vi "Begin.vi"(8 "error in":errorcluster) -> (0 "error out":errorcluster)   [LabVIEW 2019]
doc: "Called before other user functions, this VI is expected to open initial I/O refnums, load in file data, and do all program initialization. Notice that the <B>error out</B> terminal is simply used for data flow. Wiring it to other structures or subVIs ensures that this VI runs first."
uses:
  <vilib>/Rock Robotics/WPI/DriverStation/WPI_DriverStationRobotMode2.ctl
  <vilib>/Rock Robotics/WPI/Joystick/WPI_JoystickDeviceEnum.ctl
  <vilib>/Rock Robotics/WPI/SafetyOutput/WPI_SafetyOutputConfigMenu.ctl
  <vilib>/Rock Robotics/WPI/ThirdParty/REV Robotics/SPARK MAX/Typedef/Spark MAX Motor Type.ctl
  <vilib>/Rock Robotics/WPI/ThirdParty/REV Robotics/SPARK MAX/Typedef/Spark MAX Sensor Type.ctl
  <vilib>/Rock Robotics/WPI/ThirdParty/Phoenix-LabVIEW/Motor Controller/Controls/CTRE_Phoenix_MotorControl_FeedbackDevice.ctl
  <vilib>/Rock Robotics/SystemInterfaces/DIO/FPGA_DIOPWMChannel.ctl
  Robot Global Data.vi
  <vilib>/Rock Robotics/Network Tables/NT Write String Array.vi
  <vilib>/Rock Robotics/Network Tables/NT Write Number.vi
  Refnums.vi
  CAN_ID.vi
  <vilib>/Rock Robotics/WPI/RobotDrive/WPI_RobotDriveOpen2MotorWithExistingMotors.vi
  PID.vi
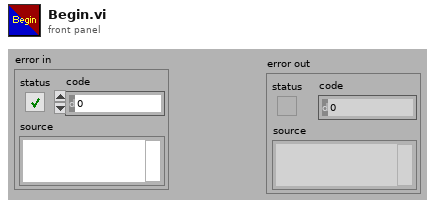
[diagram p1: front panel]
types:
  T1 = typedef "WPI_DriverStationRobotMode2.ctl" = enum16{"Autonomous Disabled", "Autonomous Enabled", "Teleop Disabled", "Teleop Enabled", "Disconnected", "Finish", "Test Disabled", "Test Enabled", "Emergency Stopped"}
  T2 = typedef "WPI_JoystickDeviceEnum.ctl" = enum16{"USB 0", "USB 1", "USB 2", "USB 3", "USB 4", "USB 5"}
  T3 = typedef "WPI_SafetyOutputConfigMenu.ctl" = enum16{"Enable", "Disable"}
  T4 = typedef "FPGA_DIOPWMChannel.ctl" = enum8{"PWM 0", "PWM 1", "PWM 2", "PWM 3", "PWM 4", "PWM 5", "PWM 6", "PWM 7", "PWM 8", "PWM 9", "PWM MXP 0", "PWM MXP 1", "PWM MXP 2", "PWM MXP 3", "PWM MXP 4", "PWM MXP 5", "PWM MXP 6", "PWM MXP 7", "PWM MXP 8", "PWM MXP 9", "Invalid"}
  T5 = typedef "WPI_JoystickDevRef.ctl" = cluster{"Device":T2}
  T6 = typedef "Spark MAX Sensor Type.ctl" = enum16{"No Sensor", "Hall Sensor", "Encoder", "-Not Available-", "Analog", "Alternate Encoder"}
  T7 = typedef "Spark MAX Motor Type.ctl" = enum16{"Brushed", "Brushless"}
  T8 = typedef "WPI_MotorControlDeviceRef.ctl" = cluster{"DeviceStatus":errorcluster, "Type":T9, "PWM":cluster{"PWM Channel":T4, "DeadBand":T10}, "CAN":cluster{"Device Number":u8, "SetOutput VI Ref":variant, "GetOutput VI Ref":variant, "Enable VI Ref":variant, "Disable VI Ref":variant, "Data":variant}, "Invert":bool, "DIO PWM":cluster{"PWM \"Enable\" Channel":T4, "DIOChannel":T11, "PWM Rate":dbl}}
  T9 = typedef "WPI_MotorControlType.ctl" = enum16{"PWM", "CAN", "DIO PWM"}
  T10 = typedef "WPI_PWMDeadband.ctl" = cluster{"Name":string, "maxPositivePwm":i32, "minPositivePwm":i32, "centerPwm":i32, "maxNegativePwm":i32, "minNegativePwm":i32, "angularRange":u16}
  T11 = typedef "FPGA_DIOChannel.ctl" = enum8{"DIO 0", "DIO 1", "DIO 2", "DIO 3", "DIO 4", "DIO 5", "DIO 6", "DIO 7", "DIO 8", "DIO 9", "DIO MXP 0", "DIO MXP 1", "DIO MXP 2", "DIO MXP 3", "DIO MXP 4", "DIO MXP 5", "DIO MXP 6", "DIO MXP 7", "DIO MXP 8", "DIO MXP 9", "DIO MXP 10", "DIO MXP 11", "DIO MXP 12", "DIO MXP 13", "DIO MXP 14", "DIO MXP 15", "SPI Port CS1", "SPI Port CS2", "SPI Port CS3", "SPI Port MISO", "SPI Port MOSI", "Invalid"}
  T12 = typedef "WPI_RobotDriveDevRef.ctl" = cluster{"DevStatus":errorcluster, "Motors[]":T8[], "Square Inputs":bool, "Max Output":dbl}
  T13 = typedef "CTRE_Phoenix_MotorControl_FeedbackDevice.ctl" = i8
  T14 = cluster{"P":dbl, "I":dbl, "D":dbl, "F":dbl, "I Zone":dbl}
  T15 = typedef "WPI_ServoDeviceRef.ctl" = cluster{"DeviceStatus":errorcluster, "PWM Channel":T4, "DeadBand":T10}
  T16 = cluster{"LEFT_FRONT_DRIVE":u8, "LEFT_REAR_DRIVE":u8, "RIGHT_FRONT_DRIVE":u8, "RIGHT_REAR_DRIVE":u8, "TALON":u8}
  T17 = cluster{"NEO_RobotDrive":T12, "TALON_SRX":T8, "RIGHT_DRIVE":T8, "LEFT_DRIVE":T8}
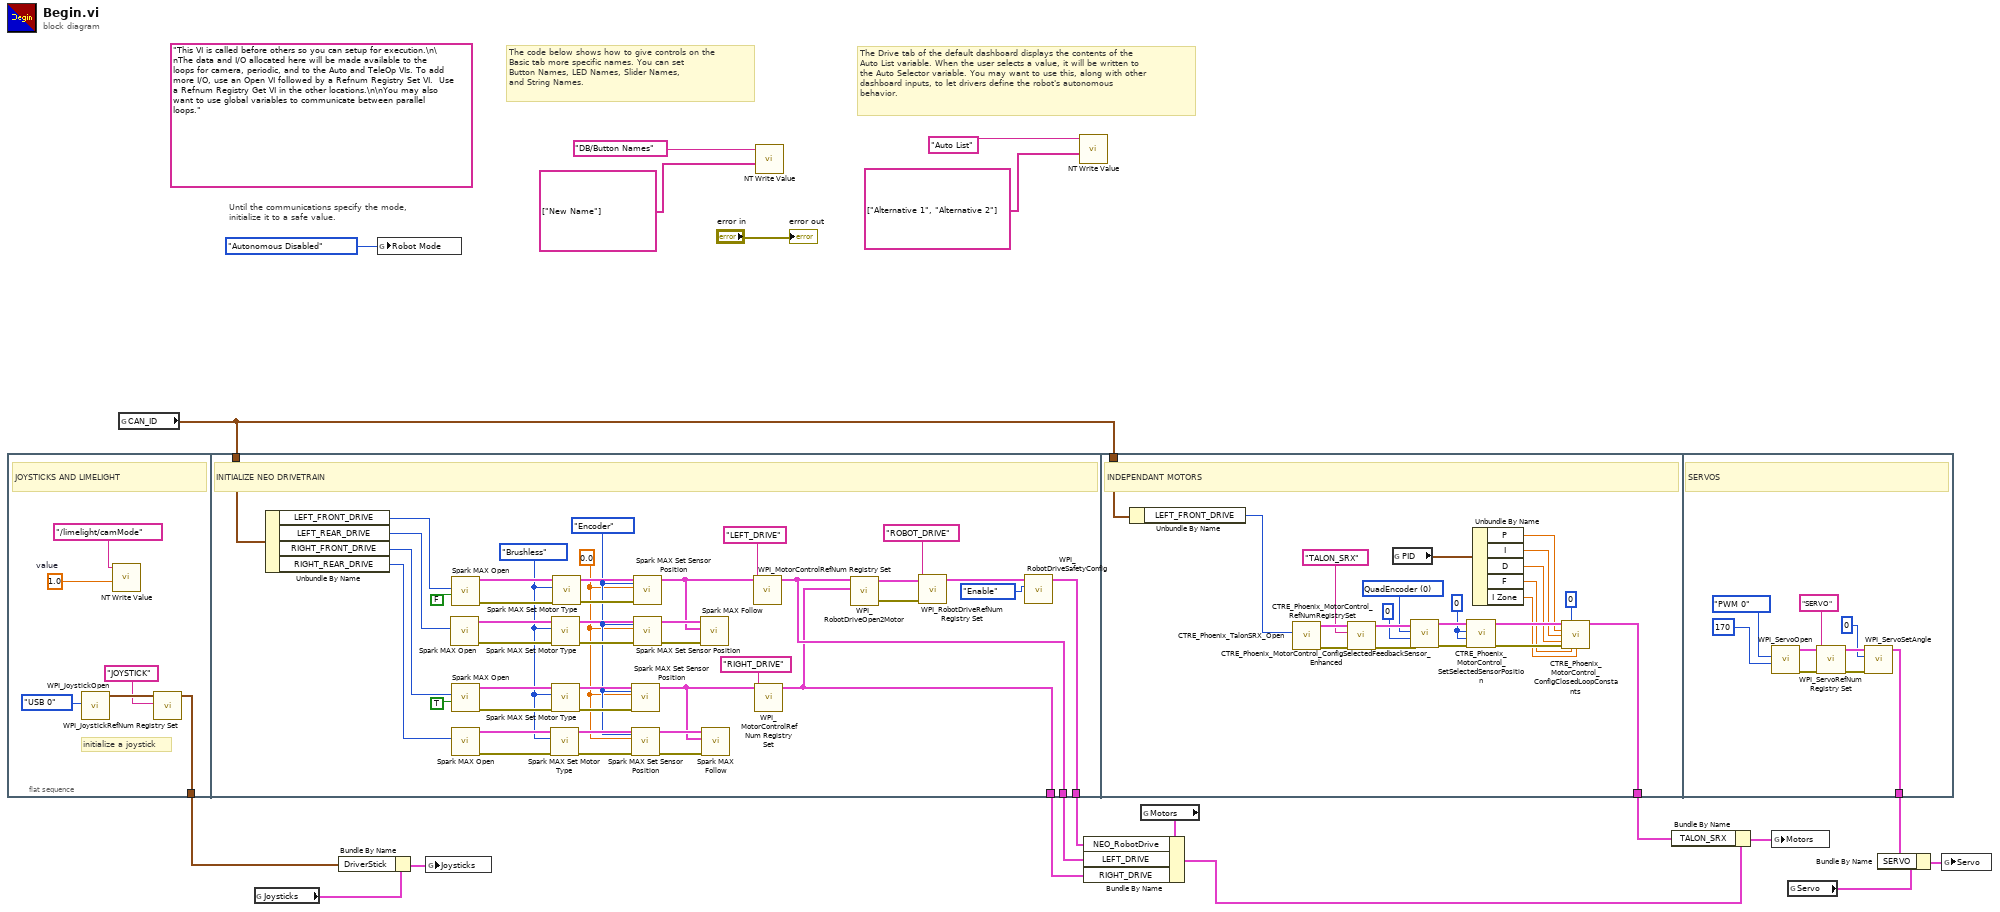
[diagram p0: block diagram]
diagram:
  (unwired) "This VI is called before others so you can setup for execution.\n\nThe data and I/O allocated here will be made available to the loops for camera, periodic, and to the Auto and TeleOp VIs. To add more I/O, use an Open VI followed by a Refnum Registry Set VI.  Use a Refnum Registry Get VI in the other locations.\n\nYou may also want to use global variables to communicate between parallel loops."
  # "The Drive tab of the default dashboard displays the contents of the\nAuto List variable. When the user selects a value, it will be written to\nthe Auto Selector variable. You may want to use this, along with other\ndashboard inputs, to let drivers define the robot's autonomous\nbehavior."
  # "The code below shows how to give controls on the\nBasic tab more specific names. You can set\nButton Names, LED Names, Slider Names,\nand String Names."
  # "Until the communications specify the mode,\ninitialize it to a safe value."
  n1 = flat-sequence {
    tunnel: [w23] -> w13
    tunnel: [w40] -> w6
    tunnel: w8 -> [w37]
    tunnel: [w28] -> w5
    tunnel: [w27] -> w4
    tunnel: [w71] -> w3
    tunnel: w8 -> [w69]
    tunnel: [w91] -> w10
    frame #0 {
      w21 = 1.0  # value
      # "initialize a joystick"
      # "JOYSTICKS AND LIMELIGHT"
      n2 = call <vilib>:"WPI_JoystickOpen.vi"("JoystickDevice"=WPI_JoystickDeviceEnum."USB 0") -> ("JoystickDevRef"=w26:T5)  [unwired: 10 in]
      n3 = call-poly <vilib>:"NT Write Value.vi"("Numeric"=w21, "Name"="/limelight/camMode") -> ()  [unwired: 9 in, 1 out]
      n4 = call <vilib>:"WPI_JoystickRefNum Registry Set.vi"("refnum name"="JOYSTICK", "JoystickDevRef"=w26) -> ("JoystickDevRef"=w23:T5)  [unwired: 8 in, 1 out]
    }
    frame #1 {
      w44 = 0.0 ("Position")
      w45 = Spark_MAX_Sensor_Type."Encoder" ("Sensor Type (Hall Sensor)")
      w43 = Spark_MAX_Motor_Type."Brushless" ("Motor Type")
      # "INITIALIZE NEO DRIVETRAIN"
      n5 = Unbundle By Name(w37) -> ("LEFT_FRONT_DRIVE"=w36:u8, "LEFT_REAR_DRIVE"=w35:u8, "RIGHT_FRONT_DRIVE"=w34:u8, "RIGHT_REAR_DRIVE"=w33:u8)
      n6 = call <vilib>:"Spark MAX Open.vi"("Device Number"=w35) -> ("error out"=w50:errorcluster, "MotorControlDeviceRef"=w49:T8)  [unwired: 9 in]
      n7 = call <vilib>:"Spark MAX Open.vi"("Invert"=FALSE, "Device Number"=w36) -> ("error out"=w48:errorcluster, "MotorControlDeviceRef"=w47:T8)  [unwired: 8 in]
      n8 = call <vilib>:"Spark MAX Open.vi"("Invert"=TRUE, "Device Number"=w34) -> ("error out"=w53:errorcluster, "MotorControlDeviceRef"=w54:T8)  [unwired: 8 in]
      n9 = call <vilib>:"Spark MAX Open.vi"("Device Number"=w33) -> ("error out"=w52:errorcluster, "MotorControlDeviceRef"=w51:T8)  [unwired: 9 in]
      n10 = call <vilib>:"Spark MAX Set Motor Type.vi"("error in (no error)"=w52, "Motor Type"=w43, "MotorControlDevRef"=w51) -> ("error out"=w62:errorcluster, "MotorControlDeviceRef"=w61:T8)  [unwired: 7 in]
      n11 = call <vilib>:"Spark MAX Set Motor Type.vi"("error in (no error)"=w50, "Motor Type"=w43, "MotorControlDevRef"=w49) -> ("error out"=w58:errorcluster, "MotorControlDeviceRef"=w57:T8)  [unwired: 7 in]
      n12 = call <vilib>:"Spark MAX Set Motor Type.vi"("error in (no error)"=w53, "Motor Type"=w43, "MotorControlDevRef"=w54) -> ("error out"=w60:errorcluster, "MotorControlDeviceRef"=w59:T8)  [unwired: 7 in]
      n13 = call <vilib>:"Spark MAX Set Motor Type.vi"("error in (no error)"=w48, "Motor Type"=w43, "MotorControlDevRef"=w47) -> ("error out"=w56:errorcluster, "MotorControlDeviceRef"=w55:T8)  [unwired: 7 in]
      n14 = call <vilib>:"Spark MAX Set Sensor Position.vi"("Sensor Type (Hall Sensor)"=w45, "error in"=w60, "Position"=w44, "MotorControlDeviceRef"=w59) -> ("MotorControlDeviceRef"=w32:T8)  [unwired: 6 in, 1 out]
      n15 = call <vilib>:"Spark MAX Set Sensor Position.vi"("Sensor Type (Hall Sensor)"=w45, "error in"=w62, "Position"=w44, "MotorControlDeviceRef"=w61) -> ("error out"=w66:errorcluster, "MotorControlDeviceRef"=w65:T8)  [unwired: 6 in]
      n16 = call <vilib>:"Spark MAX Set Sensor Position.vi"("Sensor Type (Hall Sensor)"=w45, "error in"=w56, "Position"=w44, "MotorControlDeviceRef"=w55) -> ("MotorControlDeviceRef"=w31:T8)  [unwired: 6 in, 1 out]
      n17 = call <vilib>:"Spark MAX Set Sensor Position.vi"("Sensor Type (Hall Sensor)"=w45, "error in"=w58, "Position"=w44, "MotorControlDeviceRef"=w57) -> ("error out"=w63:errorcluster, "MotorControlDeviceRef"=w64:T8)  [unwired: 6 in]
      n18 = call <vilib>:"Spark MAX Follow.vi"("error in (no error)"=w63, "Master Controller"=w31, "MotorControlDeviceRef"=w64) -> ()  [unwired: 7 in, 2 out]
      n19 = call <vilib>:"Spark MAX Follow.vi"("error in (no error)"=w66, "Master Controller"=w32, "MotorControlDeviceRef"=w65) -> ()  [unwired: 7 in, 2 out]
      n20 = call <vilib>:"WPI_MotorControlRefNum Registry Set.vi"("refnum name"="LEFT_DRIVE", "MotorControlDevRef"=w31) -> ("MotorControlDevRef"=w28:T8)  [unwired: 8 in, 1 out]
      n21 = call <vilib>:"WPI_MotorControlRefNum Registry Set.vi"("refnum name"="RIGHT_DRIVE", "MotorControlDevRef"=w32) -> ("MotorControlDevRef"=w27:T8)  [unwired: 8 in, 1 out]
      n22 = call-poly <vilib>:"WPI_RobotDriveOpen2Motor.vi"("Right Motor Dev Ref"=w27, "Left Motor Dev Ref"=w28) -> ("error out"=w68:errorcluster, "RobotDriveDevRef"=w67:T12)  [unwired: 3 in, 5 out]
      n23 = call <vilib>:"WPI_RobotDriveRefNum Registry Set.vi"("error in (no error)"=w68, "refnum name"="ROBOT_DRIVE", "RobotDriveDevRef"=w67) -> ("RobotDriveDevRef"=w46:T12)  [unwired: 1 in, 7 out]
      n24 = call <vilib>:"WPI_RobotDriveSafetyConfig.vi"("mode"=WPI_SafetyOutputConfigMenu."Enable", "RobotDriveDevRef"=w46) -> ("RobotDriveDevRef"=w40:T12)  [unwired: 8 in, 1 out]
    }
    frame #2 {
      w81 = 0 ("New Sensor Position")
      w85 = T13 0 items=["QuadEncoder"=0, "Analog"=2, "Tachometer"=4, "Pulse Width Encoded Position"=8, "Sensor Sum (S0 + S1)"=9, "Sensor Difference (D0 - D1)"=10, "Remote Source 0"=11, "Remote Source 1"=12, "Software Emulated"=15] ("Feedback Device")
      # "INDEPENDANT MOTORS"
      n25 = Unbundle By Name(w69) -> ("LEFT_FRONT_DRIVE"=w70:u8)
      n26 = call <vilib>:"CTRE_Phoenix_TalonSRX_Open.vi"("Device Number"=w70) -> ("error out"=w90:errorcluster, "CAN Talon SRX Ref"=w89:T8)  [unwired: 9 in]
      n27 = call <vilib>:"CTRE_Phoenix_MotorControl_RefNumRegistrySet.vi"("error in (no error)"=w90, "refnum name"="TALON_SRX", "PhoenixMotorControlDevRef"=w89) -> ("error out"=w87:errorcluster, "PhoenixMotorControlDevRef"=w86:T8)  [unwired: 7 in]
      n28 = global read "PID.vi" "PID"() -> (w78:T14)
      n29 = call <vilib>:"CTRE_Phoenix_MotorControl_ConfigSelectedFeedbackSensor_Enhanced.vi"("error in (no error)"=w87, "pidLoopIdx"=0, "Feedback Device"=w85, "PhoenixMotorControlDevRef"=w86) -> ("error out"=w83:errorcluster, "PhoenixMotorControlDevRef"=w82:T8)  [unwired: 6 in]
      n30 = call <vilib>:"CTRE_Phoenix_MotorControl_SetSelectedSensorPosition.vi"("error in (no error)"=w83, "pidLoopIdx"=w81, "New Sensor Position"=w81, "PhoenixMotorControlDevRef"=w82) -> ("error out"=w79:errorcluster, "PhoenixMotorControlDevRef"=w80:T8)  [unwired: 6 in]
      n31 = Unbundle By Name(w78) -> ("P"=w77:dbl, "I"=w76:dbl, "D"=w75:dbl, "F"=w74:dbl, "I Zone"=w73:dbl)
      n32 = call <vilib>:"CTRE_Phoenix_MotorControl_ConfigClosedLoopConstants.vi"("PhoenixMotorControlDevRef"=w80, "slotIdx"=0, "P"=w77, "I"=w76, "D"=w75, "error in (no error)"=w79, "F"=w74, "I Zone"=w73) -> ("PhoenixMotorControlDevRef"=w71:T8)  [unwired: 6 in, 1 out]
    }
    frame #3 {
      # "SERVOS"
      n33 = call <vilib>:"WPI_ServoOpen.vi"("Angular Range"=u16 170, "PWM Channel"=FPGA_DIOPWMChannel."PWM 0") -> ("error out"=w99:errorcluster, "ServoDeviceRef"=w98:T15)  [unwired: 8 in]
      n34 = call <vilib>:"WPI_ServoRefNum Registry Set.vi"("error in (no error)"=w99, "refnum name"="SERVO", "ServoDeviceRef"=w98) -> ("error out"=w95:errorcluster, "ServoDeviceRef"=w94:T15)  [unwired: 7 in]
      n35 = call <vilib>:"WPI_ServoSetAngle.vi"("error in (no error)"=w95, "Angle"=0, "ServoDeviceRef"=w94) -> ("ServoDeviceRef"=w91:T15)  [unwired: 7 in, 1 out]
    }
  }
  n36 = global read "CAN_ID.vi" "CAN_ID"() -> (w8:T16)
  n37 = global read "Refnums.vi" "Joysticks"() -> (w15:cluster{"DriverStick":T5, "OperatorStick":T5})
  n38 = Bundle By Name(cluster=w15, "DriverStick"=w13) -> (w12:cluster{"DriverStick":T5, "OperatorStick":T5})
  n39 = global write "Robot Global Data.vi" "Robot Mode"(WPI_DriverStationRobotMode2."Autonomous Disabled" ("Robot Mode")) -> ()
  n40 = global write "Refnums.vi" "Joysticks"(w12) -> ()
  n41 = call-poly <vilib>:"NT Write Value.vi"("String Array"=string[] ["New Name"], "Name"="DB/Button Names") -> ()  [unwired: 9 in, 1 out]
  n42 = call-poly <vilib>:"NT Write Value.vi"("String Array"=string[] ["Alternative 1", "Alternative 2"], "Name"="Auto List") -> ()  [unwired: 9 in, 1 out]
  n43 = global read "Refnums.vi" "Motors"() -> (w7:T17)
  n44 = Bundle By Name(cluster=w7, "NEO_RobotDrive"=w6, "LEFT_DRIVE"=w5, "RIGHT_DRIVE"=w4) -> (w1:T17)
  n45 = Bundle By Name(cluster=w1, "TALON_SRX"=w3) -> (w2:T17)
  n46 = global write "Refnums.vi" "Motors"(w2) -> ()
  n47 = global read "Refnums.vi" "Servo"() -> (w11:cluster{"SERVO":T15})
  n48 = Bundle By Name(cluster=w11, "SERVO"=w10) -> (w9:cluster{"SERVO":T15})
  n49 = global write "Refnums.vi" "Servo"(w9) -> ()
  "error out" <- "error in"
